vi "DrawImageWithAlphaChannel.vi"(7 "Alpha (255 opaque)":u8=255, 8 "Background Color":u32(colorbox)=16777215, 9 "Insertion Point(x,y)":cluster{"x":i16, "y":i16}, 10 "image data":T1, 11 "2D Picture in":picture) -> (3 "2D Picture out":picture)   [LabVIEW 2025, in "Picture2D.lvlib"]
uses:
  Picture2D/Picture2D.lvlib
  <vilib>/picture/picture.llb/imagedata.ctl
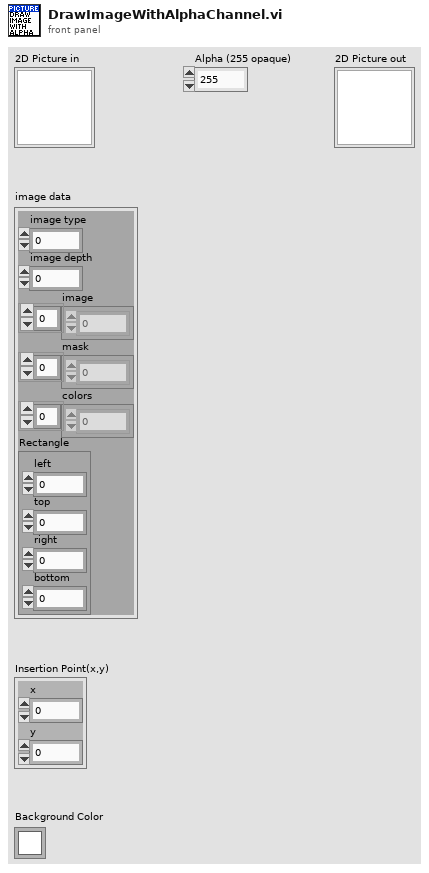
[diagram p1: front panel]
types:
  T1 = typedef "imagedata.ctl" = cluster{"image type":i32, "image depth":i32, "image":u8[], "mask":u8[], "colors":u32[], "Rectangle":cluster{"left":i16, "top":i16, "right":i16, "bottom":i16}}
  T2 = cluster{"left":i16, "top":i16, "right":i16, "bottom":i16}
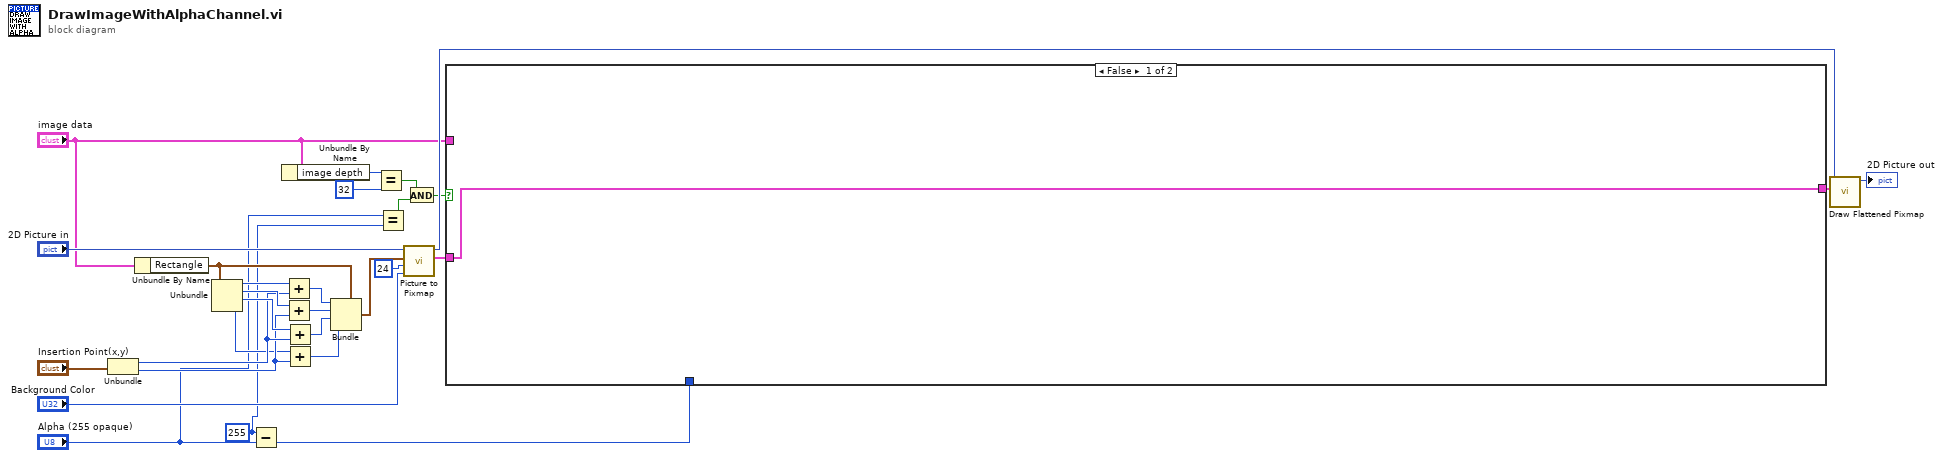
[diagram p0: block diagram]
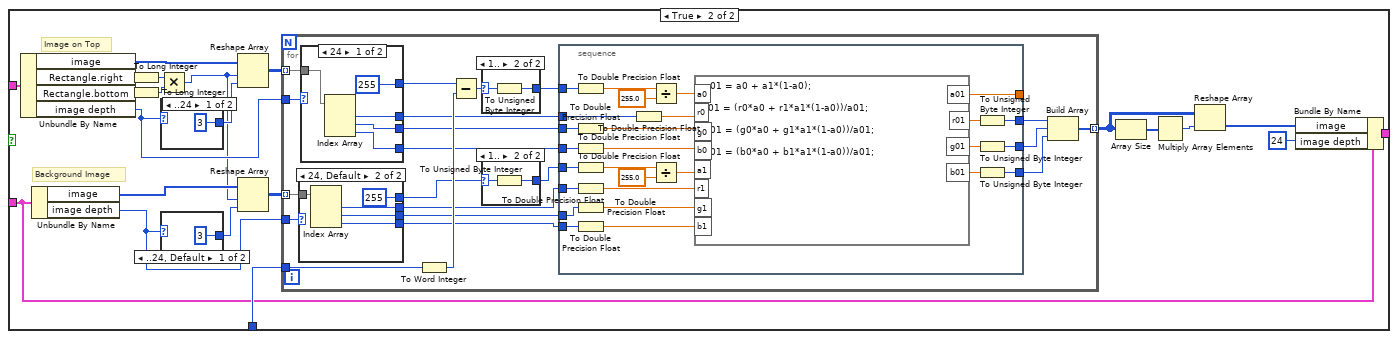
[diagram p2: hidden frame]
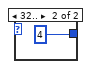
[diagram p3: hidden frame]
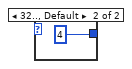
[diagram p4: hidden frame]
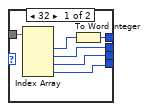
[diagram p5: hidden frame]
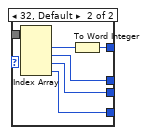
[diagram p6: hidden frame]
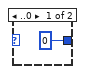
[diagram p7: hidden frame]
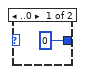
[diagram p8: hidden frame]
diagram:
  w3 = u8 255 ("x")
  n1 = Unbundle("Insertion Point(x,y)") -> ("x"=w13:i16, "y"=w12:i16)
  n2 = Unbundle By Name("image data") -> ("Rectangle"=w21:T2)
  n3 = Unbundle(w21) -> ("left"=w20:i16, "top"=w17:i16, "right"=w15:i16, "bottom"=w11:i16)
  n4 = Subtract(x=w3, y="Alpha (255 opaque)") -> (x-y=w29:u8)
  n5 = Unbundle By Name("image data") -> ("image depth"=w7:i32)
  n6 = Add(x=w20, y=w13) -> (x+y=w18:i16)
  n7 = Add(x=w17, y=w12) -> (x+y=w16:i16)
  n8 = Add(x=w15, y=w13) -> (x+y=w14:i16)
  n9 = Add(x=w11, y=w12) -> (x+y=w10:i16)
  n10 = Bundle(cluster=w21, "left"=w18, "top"=w16, "right"=w14, "bottom"=w10) -> (w9:T2)
  n11 = Equal?(x=w7, y=32) -> (x = y?=w5:bool)
  n12 = Equal?(x="Alpha (255 opaque)", y=w3) -> (x = y?=w2:bool)
  n13 = call <vilib>:"Picture to Pixmap.vi"("Background Color"="Background Color", "depth"=24, "rect"=w9, "picture"="2D Picture in") -> ("image data"=w28:T1, "new picture"=w24:picture)  [unwired: 6 in]
  n14 = And(x=w5, y=w2) -> (x .and. y?=w1:bool)
  n15 = case shown="False" w1 {
    tunnel: w29 -> [_ w52]
    tunnel: w28 -> [w30 w51]
    tunnel: "image data" -> [_ w50]
    tunnel: [w30 w40] -> w27
    frame False {
    }
    frame True {
      # "Image on Top"
      # "Background Image"
      n16 = Unbundle By Name(w50) -> ("image"=w36:u8[], "Rectangle.right"=w34:i16, "Rectangle.bottom"=w35:i16, "image depth"=w48:i32)
      n17 = Unbundle By Name(w51) -> ("image"=w38:u8[], "image depth"=w49:i32)
      n18 = To Long Integer(number=w34) -> (32bit integer=w32:i32)
      n19 = To Long Integer(number=w35) -> (32bit integer=w31:i32)
      n20 = Multiply(x=w32, y=w31) -> (x*y=w33:i32)
      n21 = case shown="..24" w48 {
        tunnel: [3 ("dimension size") 4 ("dimension size")] -> w46
        frame ..24 {
        }
        frame 32.., Default {
        }
      }
      n22 = case shown="..24, Default" w49 {
        tunnel: [3 ("dimension size") 4 ("dimension size")] -> w47
        frame ..24, Default {
        }
        frame 32.. {
        }
      }
      n23 = Reshape Array(w36, w33, w46) -> (w37:u8[][])
      n24 = Reshape Array(w38, w33, w47) -> (w39:u8[][])
      n25 = for {
        tunnel: w37 -> [w77] mode=indexing
        tunnel: w39 -> [w76] mode=indexing
        tunnel: [w75] -> w43 mode=indexing
        tunnel: w52 -> [w74]
        tunnel: w48 -> [w60]
        tunnel: w49 -> [w59]
        n26 = case shown="24, Default" w59 {
          tunnel: w76 -> [w83 w88]
          tunnel: [w82 w87] -> w66
          tunnel: [w81 w86] -> w65
          tunnel: [w80 w85] -> w64
          tunnel: [w78 i16 255] -> w58
          frame 32 {
            n27 = Index Array(array=w83) -> (element #1=w79:u8, element #2=w82:u8, element #3=w81:u8, element #4=w80:u8)  [unwired: 4 in]
            n28 = To Word Integer(number=w79) -> (16bit integer=w78:i16)
          }
          frame 24, Default {
            n29 = Index Array(array=w88) -> (element #1=w87:u8, element #2=w86:u8, element #3=w85:u8)  [unwired: 3 in]
          }
        }
        n30 = case shown="24" w60 {
          tunnel: w77 -> [w90 w99]
          tunnel: [i16 255 w97] -> w70
          tunnel: [w93 w96] -> w69
          tunnel: [w92 w95] -> w68
          tunnel: [w91 w94] -> w67
          frame 24 {
            n31 = Index Array(array=w90) -> (element #1=w93:u8, element #2=w92:u8, element #3=w91:u8)  [unwired: 3 in]
          }
          frame 32, Default {
            n32 = Index Array(array=w99) -> (element #1=w98:u8, element #2=w96:u8, element #3=w95:u8, element #4=w94:u8)  [unwired: 4 in]
            n33 = To Word Integer(number=w98) -> (16bit integer=w97:i16)
          }
        }
        n34 = To Word Integer(number=w74) -> (16bit integer=w71:i16)
        n35 = Subtract(x=w70, y=w71) -> (x-y=w73:i16)
        n36 = case shown="1.." w73 {
          selector: w73 -> [_ w132]
          tunnel: [u8 0 w131] -> w72
          frame ..0 {
          }
          frame 1.. {
            n37 = To Unsigned Byte Integer(number=w132) -> (unsigned 8bit integer=w131:u8)
          }
        }
        n38 = case shown="1.." w58 {
          selector: w58 -> [_ w102]
          tunnel: [u8 0 w101] -> w57
          frame ..0 {
          }
          frame 1.. {
            n39 = To Unsigned Byte Integer(number=w102) -> (unsigned 8bit integer=w101:u8)
          }
        }
        n40 = stacked-sequence {
          tunnel: w57 -> [w129]
          tunnel: w72 -> [w128]
          tunnel: w69 -> [w127]
          tunnel: w68 -> [w126]
          tunnel: w67 -> [w125]
          tunnel: w66 -> [w124]
          tunnel: w65 -> [w123]
          tunnel: w64 -> [w122]
          tunnel: [w121] -> w63
          tunnel: [w120] -> w62
          tunnel: [w119] -> w61
          tunnel: [w103] -> _
          frame #0 {
            n41 = To Double Precision Float(number=w128) -> (double precision float=w109:dbl)
            n42 = To Double Precision Float(number=w126) -> (double precision float=w114:dbl)
            n43 = To Double Precision Float(number=w125) -> (double precision float=w113:dbl)
            n44 = To Double Precision Float(number=w129) -> (double precision float=w105:dbl)
            n45 = To Double Precision Float(number=w124) -> (double precision float=w112:dbl)
            n46 = To Double Precision Float(number=w123) -> (double precision float=w111:dbl)
            n47 = To Double Precision Float(number=w122) -> (double precision float=w110:dbl)
            n48 = To Double Precision Float(number=w127) -> (double precision float=w115:dbl)
            n49 = Divide(x=w109, y=255.0) -> (x/y=w108:dbl)
            n50 = Divide(x=w105, y=255.0) -> (x/y=w104:dbl)
            n51 = formula code="a01 = a0 + a1*(1-a0);\n\nr01 = (r0*a0 + r1*a1*(1-a0))/a01;\n\ng01 = (g0*a0 + g1*a1*(1-a0))/a01;\n\nb01 = (b0*a0 + b1*a1*(1-a0))/a01;"("a0"=w108, "r0"=w115, "r1"=w112, "g0"=w114, "g1"=w111, "b0"=w113, "b1"=w110, "a1"=w104) -> ("r01"=w118:dbl, "g01"=w117:dbl, "b01"=w116:dbl, "a01"=w103:dbl)
            n52 = To Unsigned Byte Integer(number=w118) -> (unsigned 8bit integer=w121:u8)
            n53 = To Unsigned Byte Integer(number=w117) -> (unsigned 8bit integer=w120:u8)
            n54 = To Unsigned Byte Integer(number=w116) -> (unsigned 8bit integer=w119:u8)
          }
        }
        n55 = Build Array(w63, w62, w61) -> (w75:u8[])
      }
      n56 = Array Size(array=w43) -> (size(s)=w44:i32[])
      n57 = Multiply Array Elements(1:w44) -> (0:w45:i32)
      n58 = Reshape Array(w43, w45) -> (w42:u8[])
      n59 = Bundle By Name(cluster=w51, "image"=w42, "image depth"=24) -> (w40:T1)
    }
  }
  n60 = call <vilib>:"Draw Flattened Pixmap.vi"("image data"=w27, "picture"=w24) -> ("new picture"=→"2D Picture out":picture)  [unwired: 7 in]
